vi "Enable Disable.vi"(8 "error in (no error)":errorcluster, 11 "Node Ptr":T1 format="%.0x") -> (0 "error out":errorcluster)   [LabVIEW 2020, in "G5 Regatron Custom Device System Explorer.lvlib"]
uses:
  G5 Regatron Custom Device System Explorer.lvlib
  <vilib>/NI VeriStand/Custom Device API/Custom Device Item Ref.ctl
  Shared/Constants.vi
  <vilib>/NI VeriStand/Custom Device API/Custom Device API.lvlib
  Shared/G5 Regatron Custom Device Shared.lvlib
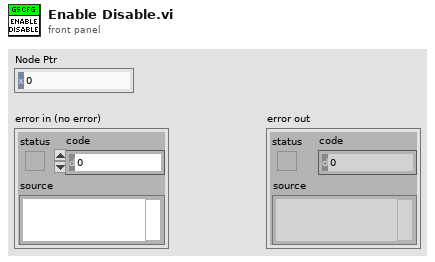
[diagram p1: front panel]
types:
  T1 = typedef "Custom Device API.lvlib/Custom Device Item Ref.ctl" = u64
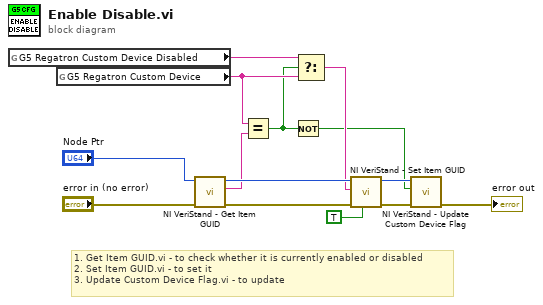
[diagram p0: block diagram]
diagram:
  # "1. Get Item GUID.vi - to check whether it is currently enabled or disabled\n2. Set Item GUID.vi - to set it\n3. Update Custom Device Flag.vi - to update"
  n1 = global read "Constants.vi" "G5 Regatron Custom Device Disabled"() -> (w5:string)
  n2 = global read "Constants.vi" "G5 Regatron Custom Device"() -> (w6:string)
  n3 = call <vilib>:"NI VeriStand - Get Item GUID.vi"("error in (no error)"="error in (no error)", "Item Ref in"="Node Ptr") -> ("error out"=w12:errorcluster, "GUID"=w7:string, "Item Ref out"=w11:T1)  [unwired: 7 in]
  n4 = Equal?(x=w6, y=w7) -> (x = y?=w4:bool)
  n5 = Not(x=w4) -> (.not. x?=w2:bool)
  n6 = Select(t=w5, s=w4, f=w6) -> (s? t:f=w3:string)
  n7 = call <vilib>:"NI VeriStand - Set Item GUID.vi"("Refresh System Explorer Tree? (F)"=TRUE, "error in (no error)"=w12, "GUID"=w3, "Item Ref in"=w11) -> ("error out"=w10:errorcluster, "Item Ref out"=w9:T1)  [unwired: 6 in]
  n8 = call <vilib>:"NI VeriStand - Update Custom Device Flag.vi"("error in (no error)"=w10, "Is Custom Device Active?"=w2, "Device Ref in"=w9) -> ("error out"=→"error out":errorcluster)  [unwired: 7 in, 1 out]
